vi "CU_splitTrainingTrials.vi"(8 "error in (no error)":errorcluster, 9 "Portion of test data":dbl=0.2 format="%#_13g", 10 "Iteration":i32 min=0 max=1 step=1, 11 "ClassifierClass in":refnum<class "ClassifierClass.lvclass">) -> (0 "error out":errorcluster, 1 "Array of Check Trials out":T1[](array[typedef]), 2 "Array of Training Trials out":T1[](array[typedef]), 3 "ClassifierClass out":refnum<class "ClassifierClass.lvclass">)   [LabVIEW 2016, in "Classifier.lvlib" / "ClassifierClass.lvclass"]
uses:
  ClassifierClass.lvclass
  _XML_EEG_Features/XML_FF_Trial.ctl
  ClassifierClass.lvclass/ClassifierClass.ctl
  _XML_EEG_Features/XML_EEG_Features.lvlib
panel:
  # "This VI is a part of BCI Design library, http://www.ru-bci.org \nCopyright © 2020, Sotnikov Peter, All rights reserved. License: GNU GPLv3"
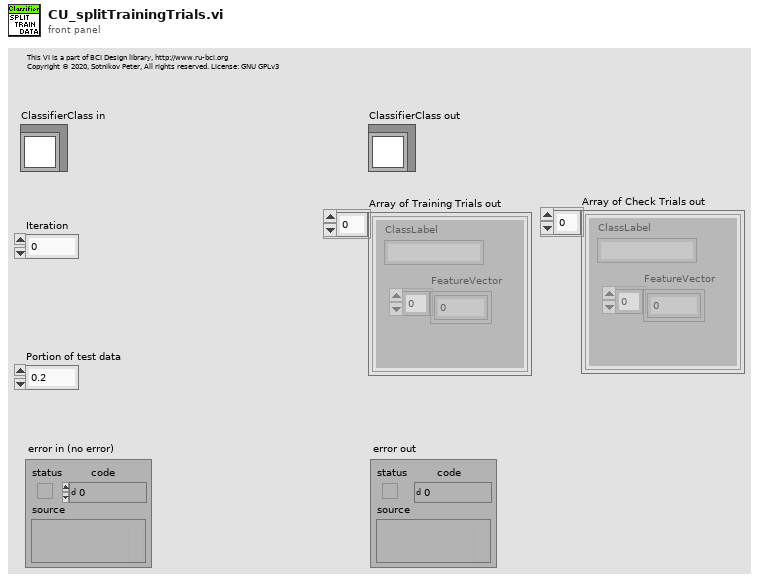
[diagram p1: front panel]
types:
  T1 = typedef "XML_EEG_Features.lvlib/XML_FF_Trial.ctl" = cluster{"ClassLabel":string, "FeatureVector":dbl[]}
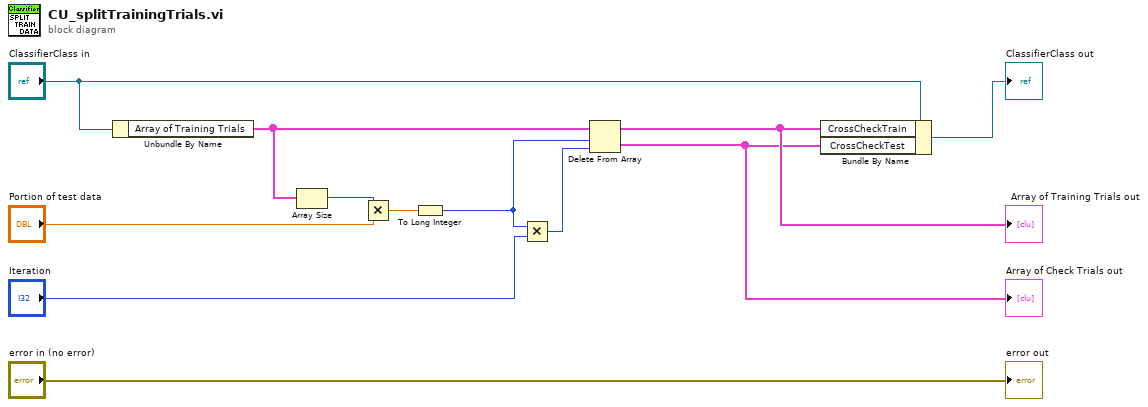
[diagram p0: block diagram]
diagram:
  n1 = Unbundle By Name("ClassifierClass in") -> ("Array of Training Trials"=w6:T1[])
  n2 = Array Size(array=w6) -> (size(s)=w7:i32)
  n3 = Multiply(x=w7, y="Portion of test data") -> (x*y=w10:dbl)
  n4 = To Long Integer(number=w10) -> (32bit integer=w4:i32)
  n5 = Multiply(x=w4, y="Iteration") -> (x*y=w2:i32)
  n6 = Delete From Array(array=w6, length=w4, index=w2) -> (deleted portion=w1:T1[], array with subset deleted=w5:T1[])
  "Array of Training Trials out" <- w5
  "Array of Check Trials out" <- w1
  n7 = Bundle By Name(cluster="ClassifierClass in", "CrossCheckTrain"=w5, "CrossCheckTest"=w1) -> (→"ClassifierClass out":refnum<class "ClassifierClass.lvclass">)
  "error out" <- "error in (no error)"
